vi "Esame.vi"() -> ()   [LabVIEW 2012]
uses:
  <vilib>/Analysis/baseanly.llb/Mean (DBL).vi
  <vilib>/Analysis/NI_AALBase.lvlib
panel:
  out "Waveform Graph":cluster{i32, "mean":dbl, dbl[][]}(graph)
  out "Media tempi":dbl format="%0.2f"
  out "output array":dbl[](array[numeric])
  out "nuova matrice A[N,15]":dbl[][](array[numeric])
  out "vettore smooting 3 elementi su n-esima riga":dbl[](array[numeric])
  out "result":dbl
  in  "Numero riga":i32
  out "n-esima riga":dbl[](array[numeric])
  out "subarray":dbl[][](array[numeric])
  out "B[N,15]":u32[][](array[numeric])
  out "A[N,15]":dbl[][](array[numeric])
  out "Tensione":string
  out "Tensione (number)":dbl
  out "x+y":u32
  out "Array N":dbl[](array[numeric])
  out "Array tempi":u32[](array[numeric])
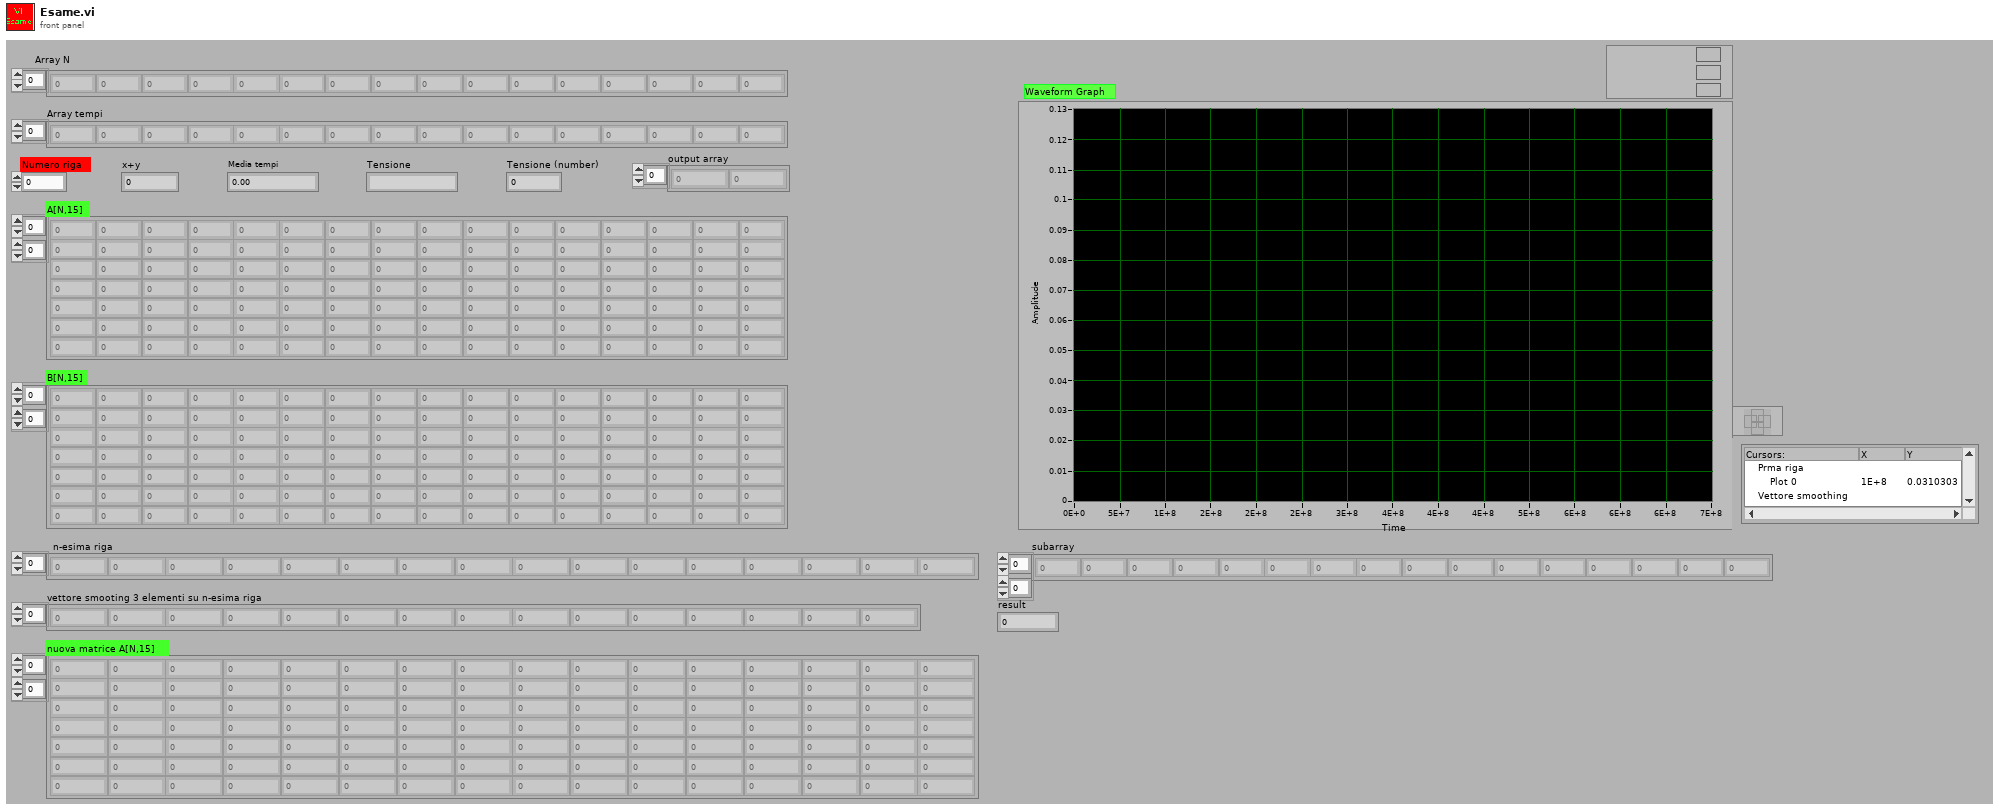
[diagram p1: front panel]
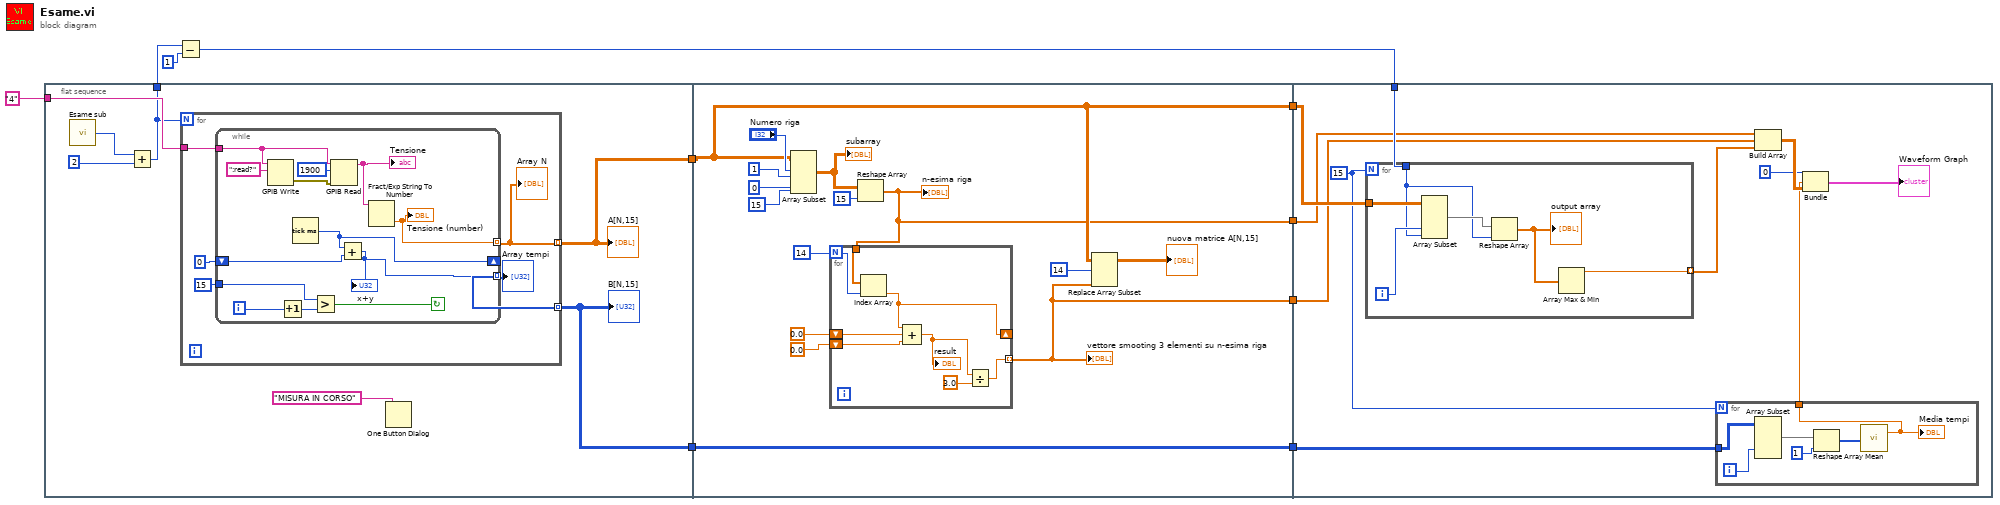
[diagram p0: block diagram]
diagram:
  n1 = flat-sequence {
    tunnel: "4" -> [w16]
    tunnel: [w14] -> w3
    tunnel: [w12] -> w9
    tunnel: [w11] -> w5
    tunnel: w9 -> [w43]
    tunnel: [w43] -> w8
    tunnel: [w44] -> w7
    tunnel: [w41] -> w6
    tunnel: w5 -> [w40]
    tunnel: [w40] -> w4
    tunnel: w8 -> [w69]
    tunnel: w7 -> [w66]
    tunnel: w6 -> [w65]
    tunnel: w4 -> [w64]
    tunnel: w1 -> [w68]
    frame #0 {
      n2 = call "Esame sub.vi"() -> ("N"=w15:i32)
      n3 = Add(x=w15, y=2) -> (x+y=w14:i32)
      n4 = for {
        N: w14 -> [_]
        tunnel: w16 -> [w22]
        tunnel: [w20] -> w12 mode=indexing
        tunnel: [w18] -> w11 mode=indexing
        n5 = while {
          tunnel: 15 -> [w33]
          tunnel: w22 -> [w30]
          tunnel: [w26] -> w20 mode=indexing
          shift-right: [w24] -> _
          shift-left: u32 0 -> [w25]
          tunnel: [w23] -> w18 mode=indexing
          i -> [w35]
          stop <- w32 continue-if-true
          n6 = GPIB Write(0:w30, 1:":read?" ("data")) -> (6:w28:errorcluster)  [unwired: 3 in, 1 out]
          n7 = Increment(x=w35) -> (x+1=w34:i32)
          n8 = Tick Count (ms)() -> (millisecond timer value=w24:u32)
          n9 = Greater?(x=w33, y=w34) -> (0:w32:bool)
          n10 = GPIB Read(0:w30, 1:1900 ("byte count"), 3:w28) -> (5:w27:string)  [unwired: 2 in, 2 out]
          "Tensione" <- w27
          n11 = Add(x=w24, y=w25) -> (x+y=w23:u32)
          "x+y" <- w23
          n12 = Fract/Exp String To Number(string=w27) -> (number=w26:dbl)  [unwired: 3 in, 1 out]
          "Tensione (number)" <- w26
        }
        "Array N" <- w20
        "Array tempi" <- w18
      }
      "A[N,15]" <- w12
      "B[N,15]" <- w11
      n13 = One Button Dialog(message="MISURA IN CORSO") -> ()  [unwired: 1 in, 1 out]
    }
    frame #1 {
      n14 = Array Subset(array=w43, index (row)="Numero riga", length (row)=1 ("length"), index (col)=0 ("index"), length (col)=15 ("length")) -> (w47:dbl[][])
      "subarray" <- w47
      n15 = Reshape Array(w47, 15 ("dimension size")) -> (w41:dbl[])
      "n-esima riga" <- w41
      n16 = for {
        N: 14 -> [w51]
        tunnel: w41 -> [w58]
        shift-right: [w52] -> _
        shift-left: 0.0 -> [w57]
        shift-left: 0.0 -> [w56]
        tunnel: [w53] -> w44 mode=indexing
        n17 = Index Array(array=w58, index=w51) -> (element=w52:dbl)
        n18 = Compound Arithmetic op=ADD(w52, w57, w56) -> (w54:dbl)
        "result" <- w54
        n19 = Divide(x=w54, y=3.0) -> (x/y=w53:dbl)
      }
      "vettore smooting 3 elementi su n-esima riga" <- w44
      n20 = Replace Array Subset(array=w43, new element=w44, index (row)=14) -> (→"nuova matrice A[N,15]":dbl[][])  [unwired: 1 in]
    }
    frame #2 {
      w63 = 15
      n21 = for {
        N: w63 -> [_]
        tunnel: [w78] -> w67 mode=indexing
        tunnel: w69 -> [w77]
        tunnel: w68 -> [w76]
        i -> [w81]
        n22 = Array Subset(array=w77, index (col)=w81, length (col)=w76) -> (w80:dbl[][])  [unwired: 2 in]
        n23 = Reshape Array(w80, w76) -> (w79:dbl[])
        "output array" <- w79
        n24 = Array Max & Min(array=w79) -> (max value=w78:dbl)  [unwired: 3 out]
      }
      n25 = for {
        N: w63 -> [_]
        tunnel: w64 -> [w72]
        tunnel: [w70] -> w60
        i -> [w71]
        n26 = Array Subset(array=w72, index (col)=w71) -> (w75:u32[][])  [unwired: 3 in]
        n27 = Reshape Array(w75, 1 ("dimension size")) -> (w74:u32[])
        n28 = call-poly <vilib>:"Mean.vi"("X"=w74) -> ("mean"=w70:dbl)  [unwired: 1 out]
        "Media tempi" <- w70
      }
      n29 = Build Array(w65, w66, w67) -> (w62:dbl[][])
      n30 = Bundle(0, "mean"=w60, w62) -> (→"Waveform Graph":cluster{i32, "mean":dbl, dbl[][]})  [unwired: 1 in]
    }
  }
  n31 = Subtract(x=w3, y=1) -> (x-y=w1:i32)
